vi "wpisywanie tekstu do pliku txt.vi"() -> ()   [LabVIEW 2017]
panel:
  out "error in":errorcluster
  in  "file path (use dialog)":path
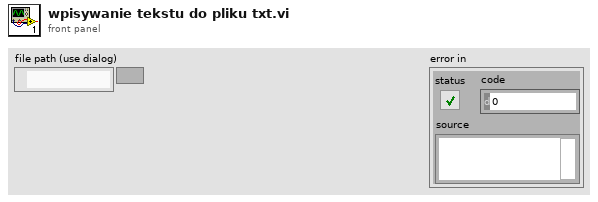
[diagram p1: front panel]
types:
  T1 = enum16{"open", "replace", "create", "open or create", "replace or create", "replace or create with confirmation"}
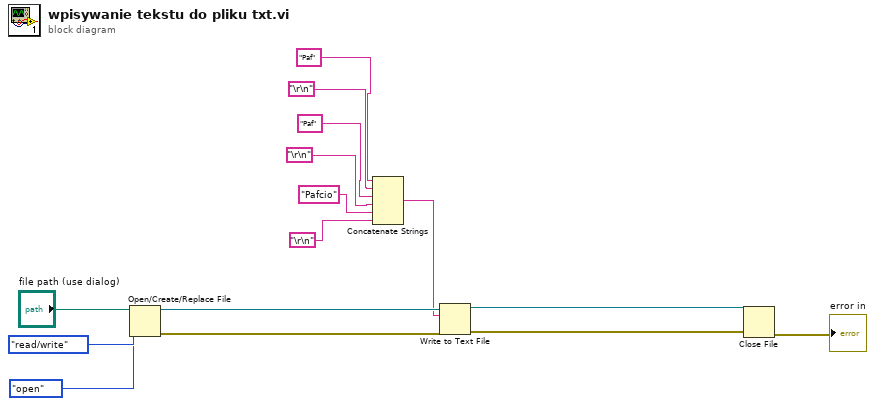
[diagram p0: block diagram]
diagram:
  n1 = Open/Create/Replace File(file path (use dialog)="file path (use dialog)", operation (0:open)=T1."open", access (0:read/write)=enum16{"read/write", "read-only", "write-only"}."read/write") -> (refnum out=w14:refnum<file>, error out=w12:errorcluster)  [unwired: 3 in, 1 out]
  n2 = Concatenate Strings("Paf", "\r\n", "Paf", "\r\n", "Pafcio", "\r\n") -> (w10:string)
  n3 = Write to Text File(file (use dialog)=w14, text=w10, error in=w12) -> (refnum out=w13:refnum<file>, error out=w11:errorcluster)  [unwired: 1 in, 1 out]
  n4 = Close File(refnum=w13, error in=w11) -> (error out=→"error in":errorcluster)  [unwired: 1 out]
